vi "fg_event.vi"(8 "error in (no error)":errorcluster) -> (0 "error out":errorcluster, 2 "data":T1, 3 "launcher_event":refnum<user-event>)   [LabVIEW 2015, in "lv-launcher-nre.lvlib"]
uses:
  lv-launcher-nre.lvlib
  _controls/event.ctl
  _controls/event_command.ctl
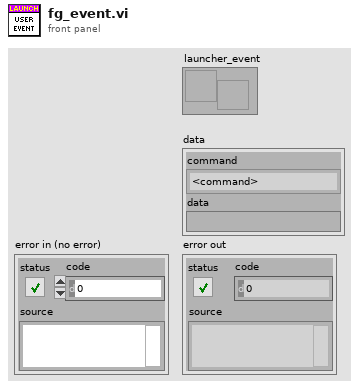
[diagram p1: front panel]
types:
  T1 = typedef "lv-launcher-nre.lvlib/event.ctl" = cluster{"command":T2, "data":variant}
  T2 = typedef "lv-launcher-nre.lvlib/event_command.ctl" = enum16{"<command>", "die", "<null>"}
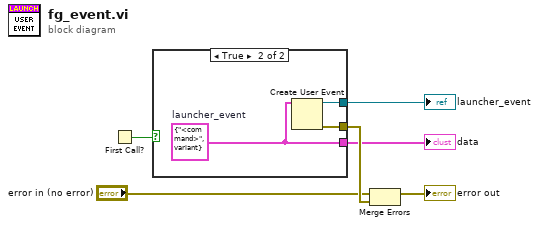
[diagram p0: block diagram]
diagram:
  n1 = First Call?() -> (First Call?: T/F=w4:bool)
  n2 = case shown="True" w4 {
    tunnel: [_ w9] -> w1
    tunnel: [_ w8] -> w6
    tunnel: [_ w7] -> w5
    frame False {
    }
    frame True {
      w7 = T1 {"command"=enum."<command>", "data"=variant}  # launcher_event
      n3 = Create User Event(user event datatype=w7) -> (user event=w9:refnum<user-event>, error out=w8:errorcluster)  [unwired: 1 in]
    }
  }
  "data" <- w5
  "launcher_event" <- w1
  n4 = Merge Errors("error in (no error)", w6) -> (→"error out":errorcluster)
